vi "Sine Curve Fitting.vi"() -> ()   [LabVIEW 2023]
doc: "The example shows the application of the adaptive transform in detecting parameters of a sine wave. \n\nYou can use many methods to detect the parameters (offset, amplitude, phase, and frequency) of a sine wave. For example, you can use the power spectrum to estimate the frequency of the sine wave and then use correlation to detect the amplitude and phase. However, the resolution of this method is limited by the number of samples in the signal. The adaptive transform based method applies a Gaussian window to the sine wave to form a Gaussian pulse signal, uses the adaptive transform to detect the frequency and phase of the sine wave, and finally uses linear-fitting to estimate the amplitude and offset of the sine wave. The adaptive transform-based method has high frequency resolution. Moreover, you also can use this method to detect parameters of multi-tone signals.\n\nThis example first uses the TFA Adaptive Transform VI to detect the frequencies and phases of sine waves, then computes the amplitudes and offsets of the sine waves by linear-fitting.\n\n<b>Instructions:</b>\n1) Run this VI.\n2) Observe the <b>Detected Frequencies</b> of the signal.\n3) Change the settings of the simulated signal and observe the detected results.\n4) Browse the Block Diagram to learn how to implement sine wave fitting with adaptive transform."
uses:
  <vilib>/addons/Time Frequency Analysis/Transform.llb/TFA Adaptive Transform (Waveform).vi
  <vilib>/measure/NI_MABase.lvlib
  <vilib>/addons/_Advanced Signal Processing/NI_AdvSigProcTFA.lvlib
  <vilib>/measure/NI_MAPro.lvlib
panel:
  out "aspt-left-top":bool
  in  "Stop":bool
  in  "Noise amplitude":dbl=1.0
  out "Reconstructed Signal":waveform(dbl)(graph)
  out "Detected frequencies":dbl[](array[numeric]) format="%.2f"
  in  "Frequencies":dbl[](array[numeric])=[30.0, 40.0] format="%.2f"
  out "Multiple Sine Waves with Noise":waveform(dbl)(graph)
  # "Overview: Shows the application of the adaptive transform in detecting parameters of a sine wave.\nRequirements: LabVIEW Full Development System, Advanced Signal Processing Toolkit\nInstructions: \n1. Run this VI.\n2. Observe the Detected Frequencies of the signal.\n3. Change the settings of the simulated signal and observe the detected results.\n4. Browse the block diagram to learn how to implement sine wave fitting with adaptive transform.\n5. Click Stop to stop the VI."
  # "Simulated Signal"
  # "Detected Tones"
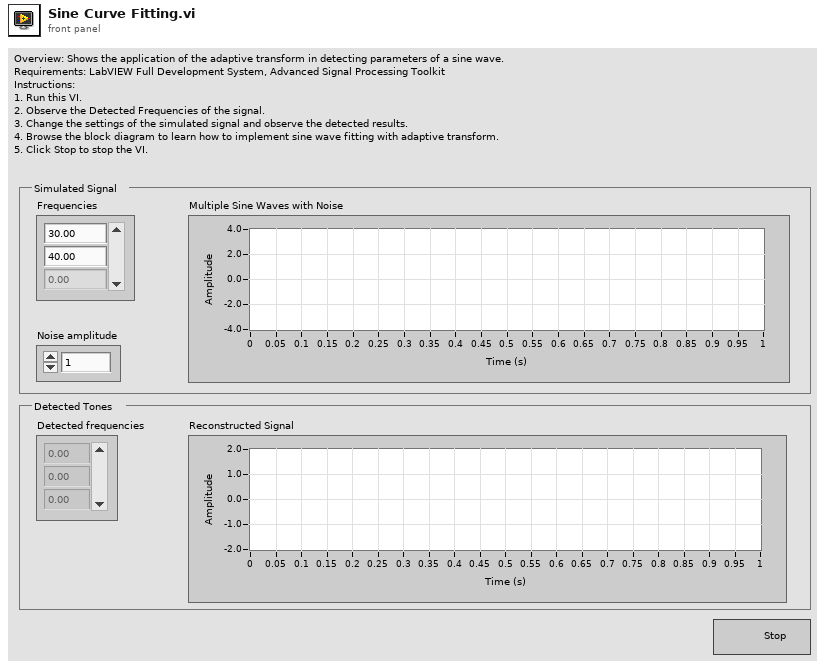
[diagram p1: front panel]
types:
  T1 = cluster{"type":u16, "max window length":i32, "reserved":i32}
  T2 = cluster{"amplitude":cdb, "standard deviation":dbl, "center":dbl, "frequency":dbl, "chirp rate":dbl}[]
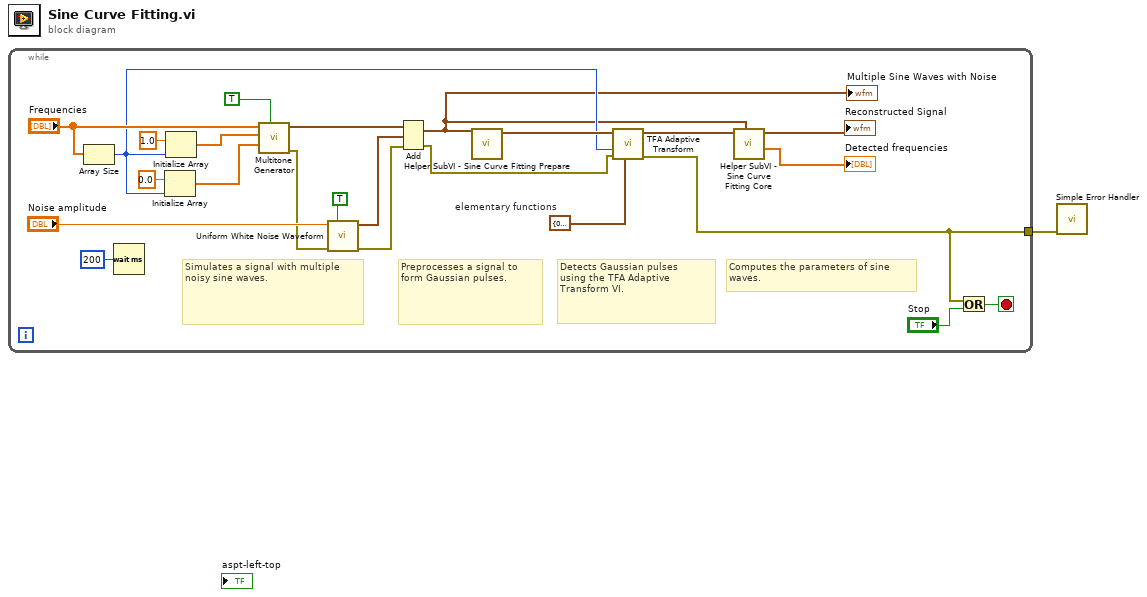
[diagram p0: block diagram]
diagram:
  n1 = while {
    tunnel: [w2] -> w1
    stop <- w8 stop-if-true
    w11 = T1 {"type"=0, "max window length"=-1, "reserved"=-1}  # elementary functions
    # "Computes the parameters of sine waves."
    # "Detects Gaussian pulses\nusing the TFA Adaptive Transform VI."
    # "Preprocesses a signal to \nform Gaussian pulses."
    # "Simulates a signal with multiple \nnoisy sine waves."
    n2 = Array Size(array="Frequencies") -> (size(s)=w15:i32)
    n3 = Wait (ms)(milliseconds to wait=u32 200 ("millisecond multiple")) -> ()  [unwired: 1 out]
    n4 = Initialize Array(0.0 ("element"), w15) -> (w17:dbl[])
    n5 = Initialize Array(1.0 ("element"), w15) -> (w16:dbl[])
    n6 = call <vilib>:"Multitone Generator.vi"("reset signal"=TRUE, "tone phases"=w17, "tone amplitudes"=w16, "tone frequencies"="Frequencies") -> ("error out"=w3:errorcluster, "signal out"=w21:waveform(dbl))  [unwired: 4 in, 2 out]
    n7 = call <vilib>:"Uniform White Noise Waveform.vi"("reset signal"=TRUE, "error in (no error)"=w3, "amplitude"="Noise amplitude") -> ("error out"=w5:errorcluster, "signal out"=w25:waveform(dbl))  [unwired: 2 in, 5 out]
    n8 = Add(1:w25, 2:w21, 4:w5) -> (0:w14:waveform(dbl), 3:w4:errorcluster)
    "Multiple Sine Waves with Noise" <- w14
    n9 = call "Helper SubVI - Sine Curve Fitting Prepare.vi"("signal in"=w14) -> ("signal out"=w23:waveform(dbl))  [unwired: 10 in]
    n10 = call-poly <vilib>:"TFA Adaptive Transform.vi"("elementary functions"=w11, "error in (no error)"=w4, "number of terms"=w15, "signal"=w23) -> ("error out"=w2:errorcluster, "chirplet info"=w24:T2)  [unwired: 6 out]
    n11 = call "Helper SubVI - Sine Curve Fitting Core.vi"("signal in"=w14, "ADT paras"=w24) -> ("Frequencies"=→"Detected frequencies":dbl[], "signal out"=→"Reconstructed Signal":waveform(dbl))  [unwired: 8 out]
    n12 = Or(x=w2, y="Stop") -> (x .or. y?=w8:bool)
  }
  n13 = call <vilib>:"Simple Error Handler.vi"("error in (no error)"=w1) -> ()  [unwired: 1 in, 8 out]
